vi "ScanForDevices.vi"(8 "Error in":errorcluster, 9 "SortedBy":i32(ring) items=["Serialnumber", "Name", "IpAddress"], 11 "AvailableDeviceFamilies":string[](array[string])) -> (0 "Error out":errorcluster, 3 "Devices":refnum<k24>[](array[refnum]))   [LabVIEW 2016]
doc: "Scans for devices. Repeat this several times to find more devices.\nNotice: Typically you have to wait 6 seconds after the execution of the Init.vi until all devices that support the scan mechanism are collected and will be returned by this VI. So if you want to use the Scan.vi only once (e.g. within a non-interactive workflow), you have to assert that 6 seconds passed since executing the Init.vi to be sure to get all available devices.\n\nAvailableDeviceFamilies: Array of device family names (e.g. PMX, QuantumX) you want to scan. Leave this connection empty to find all scanable devices of all device families.\nSortedBy: Enumeration that defines the property (Name, IpAddress or SerialNumber) that will be used to sort the found devices.\nDevices: Found and sorted devices according to given device family names and sorting settings."
uses:
  C:/Users/CL/Desktop/ZcDAQprj0811/ZcDAQprj/Modules/DAQ-Device/Hardware Drivers/QX/HBM LabVIEW Driver/DLLs/Hbm.Api.Common.dll
  DLLs/Hbm.Api.Common.dll
  C:/Users/CL/Desktop/ZcDAQprj0811/ZcDAQprj/Modules/DAQ-Device/Hardware Drivers/QX/HBM LabVIEW Driver/DLLs/Hbm.Api.LabVIEW.dll
  DLLs/Hbm.Api.LabVIEW.dll
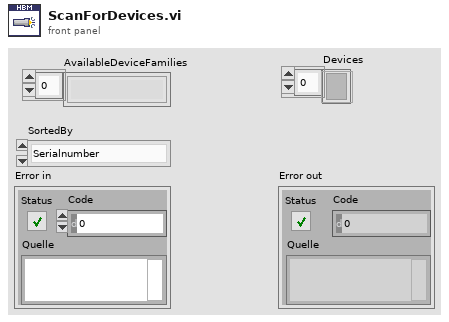
[diagram p1: front panel]
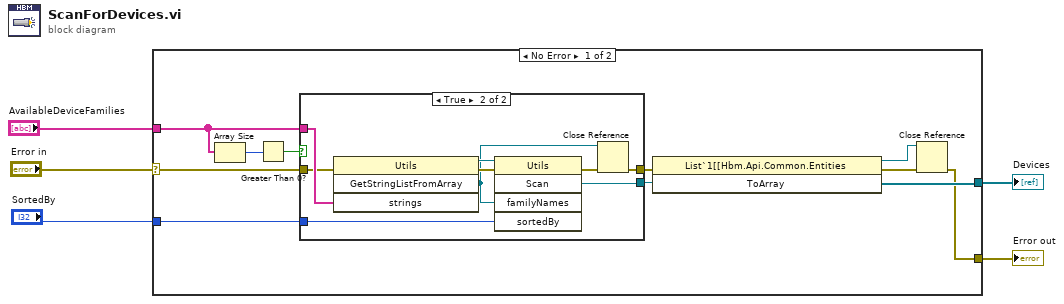
[diagram p0: block diagram]
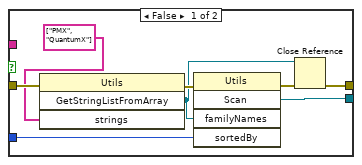
[diagram p2: hidden frame]
diagram:
  n1 = case shown="No Error" "Error in" {
    selector: "Error in" -> [w10 w34]
    tunnel: [w6 w34] -> w4
    tunnel: "AvailableDeviceFamilies" -> [w14 _]
    tunnel: [w11 _] -> w2
    tunnel: "SortedBy" -> [w9 _]
    frame No Error {
      n2 = Array Size(array=w14) -> (size(s)=w16:i32)
      n3 = Greater Than 0?(x=w16) -> (x > 0?=w15:bool)
      n4 = case shown="True" w15 {
        tunnel: [w18 w26] -> w12
        tunnel: w14 -> [_ w33]
        tunnel: [w24 w30] -> w13
        tunnel: w10 -> [w23 w32]
        tunnel: w9 -> [w20 w28]
        frame False {
          n5 = invoke on="Methodenknoten" class="Utils" method="GetStringListFromArray"(error in=w23, "strings"=string[] ["PMX", "QuantumX"] ("AvailableDeviceFamilies")) -> (error out=w22:errorcluster, "GetStringListFromArray"=w17:refnum<k24>)  [unwired: 2 in, 2 out]
          n6 = invoke on="Methodenknoten" class="Utils" method="Scan"(error in=w22, "familyNames"=w17, "sortedBy"=w20) -> (error out=w19:errorcluster, "Scan"=w24:refnum<k24>)  [unwired: 2 in, 3 out]
          n7 = Close Reference(reference=w17, error in (no error)=w19) -> (error out=w18:errorcluster)
        }
        frame True {
          n8 = invoke on="Methodenknoten" class="Utils" method="GetStringListFromArray"(error in=w32, "strings"=w33) -> (reference out=w31:refnum<k24>, error out=w29:errorcluster, "GetStringListFromArray"=w25:refnum<k24>)  [unwired: 2 in, 1 out]
          n9 = invoke on="Methodenknoten" class="Utils" method="Scan"(reference=w31, error in=w29, "familyNames"=w25, "sortedBy"=w28) -> (error out=w27:errorcluster, "Scan"=w30:refnum<k24>)  [unwired: 1 in, 3 out]
          n10 = Close Reference(reference=w25, error in (no error)=w27) -> (error out=w26:errorcluster)
        }
      }
      n11 = invoke class="List`1[[Hbm.Api.Common.Entities" method="ToArray"(reference=w13, error in=w12) -> (reference out=w7:refnum<k24>, error out=w8:errorcluster, "ToArray"=w11:refnum<k24>[])  [unwired: 1 in]
      n12 = Close Reference(reference=w7, error in (no error)=w8) -> (error out=w6:errorcluster)
    }
    frame Error {
    }
  }
  "Error out" <- w4
  "Devices" <- w2
